vi "ASI.vi"(4 "Special Function In":string, 6 "Velocity":dbl, 7 "Abort":refnum<vi>, 8 "Axis":bool[](array[boolean]), 9 "Positions In":dbl[](array[numeric]), 10 "Action":T1=enum."MVR", 11 "VISA In":refnum<visa-resource-name>) -> (0 "Special Function Out":string, 1 "Status":bool, 2 "Position Out":dbl[](array[numeric]), 3 "VISA Out":refnum<visa-resource-name>)   [LabVIEW 2014]
uses:
  Controls/StageStates.ctl
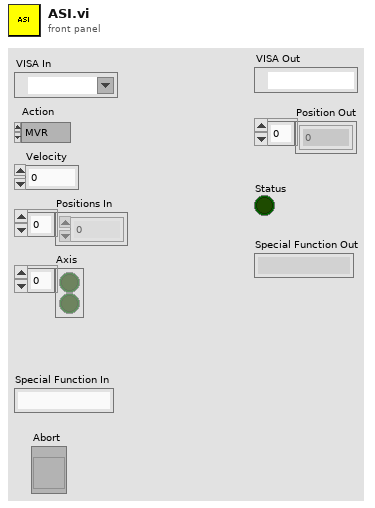
[diagram p1: front panel]
types:
  T1 = typedef "StageStates.ctl" = enum16{"POSITION", "MVR", "MOVE", "HALT", "ONTARGET", "ERROR", "EXIT", "HOME", "ZEROPOS", "NANOPOS", "QUIT", "ANALOG"}
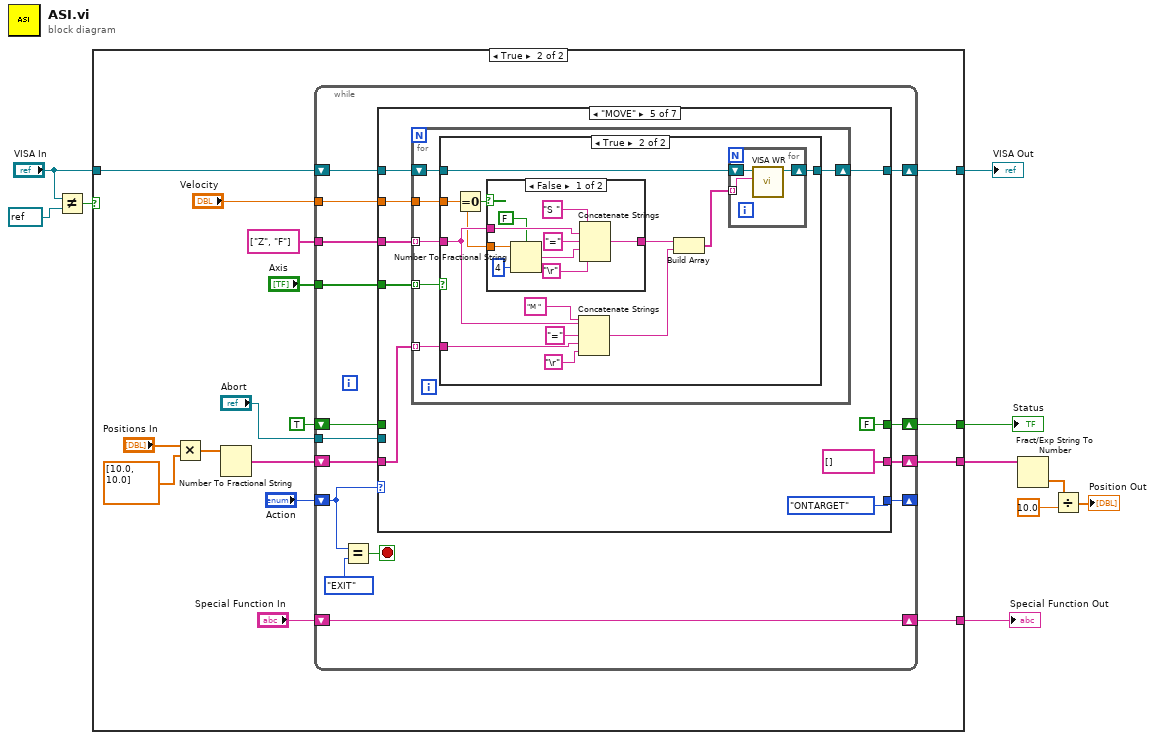
[diagram p0: block diagram]
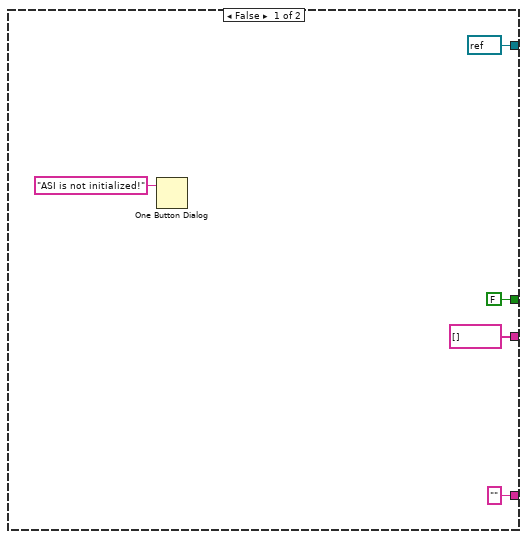
[diagram p2: hidden frame]
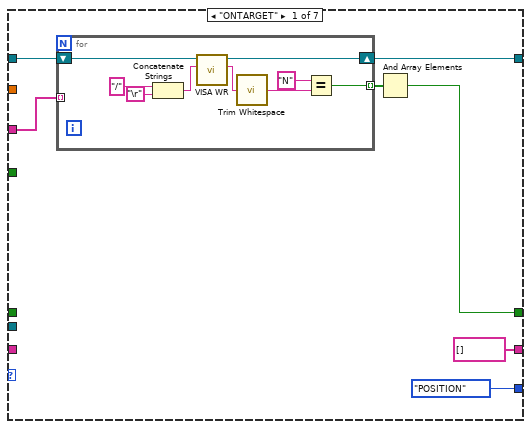
[diagram p3: hidden frame]
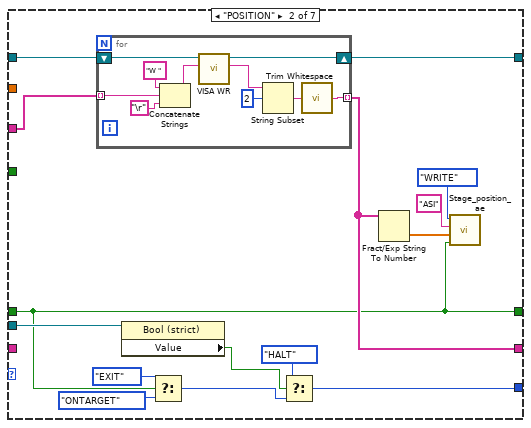
[diagram p4: hidden frame]
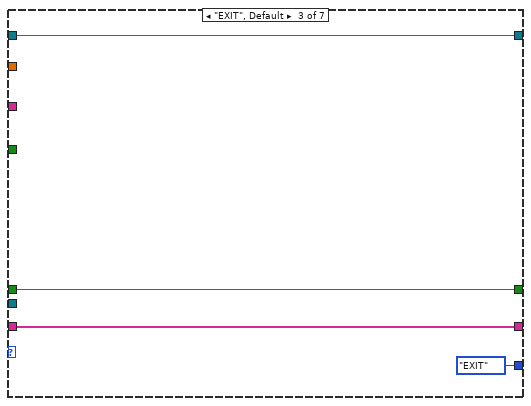
[diagram p5: hidden frame]
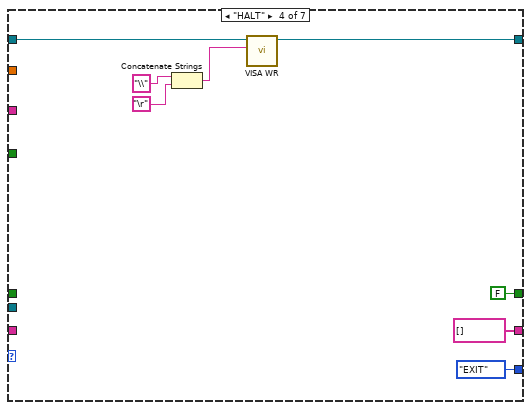
[diagram p6: hidden frame]
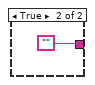
[diagram p8: hidden frame]
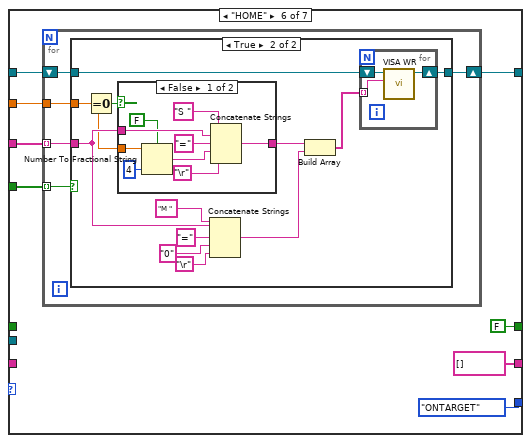
[diagram p9: hidden frame]
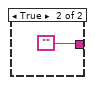
[diagram p11: hidden frame]
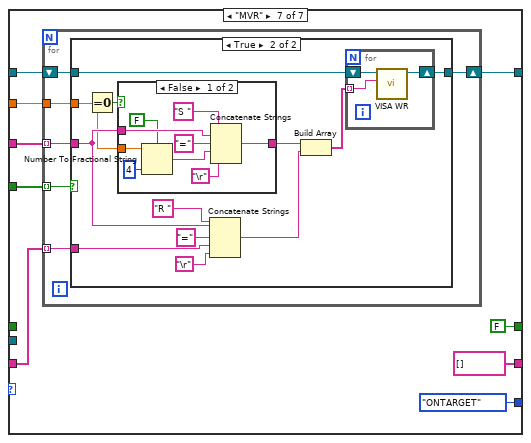
[diagram p12: hidden frame]
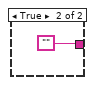
[diagram p14: hidden frame]
diagram:
  n1 = Not Equal?(x="VISA In", y=refnum<visa-resource-name> refnum ("VISA resource name")) -> (x != y?=w8:bool)
  n2 = case shown="True" w8 {
    tunnel: "VISA In" -> [_ w30]
    tunnel: [refnum<visa-resource-name> refnum ("VISA In") w23] -> w4
    tunnel: [FALSE w22] -> w3
    tunnel: [string[] [] w21] -> w2
    tunnel: ["" ("Special Function In") w20] -> w1
    frame False {
      n3 = One Button Dialog(message="ASI is not initialized!") -> ()  [unwired: 1 in, 1 out]
    }
    frame True {
      n4 = Multiply(x="Positions In", y=dbl[] [10.0, 10.0]) -> (x*y=w16:dbl[])
      n5 = Number To Fractional String(number=w16) -> (F-format string=w25:string[])  [unwired: 3 in]
      n6 = while {
        tunnel: string[] ["Z", "F"] -> [w46]
        shift-right: [w35] -> _
        shift-left: "Action" -> [w40]
        shift-right: [w43] -> w21
        shift-left: w25 -> [w44]
        shift-right: [w41] -> w22
        shift-left: TRUE -> [w42]
        tunnel: "Axis" -> [w39]
        tunnel: "Velocity" -> [w38]
        shift-right: [w37] -> w20
        shift-left: "Special Function In" -> [w37]
        shift-right: [w33] -> w23
        shift-left: w30 -> [w45]
        tunnel: "Abort" -> [w32]
        stop <- w34 stop-if-true
        n7 = Equal?(x=w40, y=StageStates."EXIT") -> (x = y?=w34:bool)
        n8 = case shown="\"MOVE\"" w40 {
          tunnel: w46 -> [w50 w76 _ _ w108 w148 w188]
          tunnel: w45 -> [w53 w77 w88 w99 w107 w147 w187]
          tunnel: w44 -> [_ _ w90 _ w106 _ w186]
          tunnel: [string[] [] w75 w90 string[] [] string[] [] string[] [] string[] []] -> w43
          tunnel: w42 -> [_ w64 w91 _ _ _ _]
          tunnel: [w51 w64 w91 FALSE FALSE FALSE FALSE] -> w41
          tunnel: w39 -> [_ _ _ _ w105 w146 w185]
          tunnel: w38 -> [_ _ _ _ w104 w145 w184]
          tunnel: [StageStates."POSITION" ("Action") w69 StageStates."EXIT" ("Action") StageStates."EXIT" ("Action") StageStates."ONTARGET" ("Action") StageStates."ONTARGET" ("Action") StageStates."ONTARGET" ("Action")] -> w35
          tunnel: [w47 w67 w88 w92 w100 w141 w180] -> w33
          tunnel: w32 -> [_ w65 _ _ _ _ _]
          frame "ONTARGET" {
            n9 = for {
              tunnel: [w58] -> w52 mode=indexing
              tunnel: w50 -> [_] mode=indexing
              shift-right: [w54] -> w47
              shift-left: w53 -> [w62]
              n10 = Concatenate Strings("/" ("string"), "\r") -> (w61:string)
              n11 = call "VISA WR.vi"("write buffer"=w61, "VISA Refnum in"=w62) -> ("read buffer"=w60:string, "VISA Refnum out"=w54:refnum<visa-resource-name>)  [unwired: 7 in, 1 out]
              n12 = call <vilib>:"Trim Whitespace.vi"("string"=w60) -> ("trimmed string"=w55:string)  [unwired: 1 in]
              n13 = Equal?(x="N", y=w55) -> (x = y?=w58:bool)
            }
            n14 = And Array Elements(Boolean array=w52) -> (logical AND=w51:bool)
          }
          frame "POSITION" {
            n15 = for {
              tunnel: [w84] -> w75 mode=indexing
              tunnel: w76 -> [w79] mode=indexing
              shift-right: [w78] -> w67
              shift-left: w77 -> [w87]
              n16 = Concatenate Strings("W " ("string"), w79, "\r") -> (w86:string)
              n17 = call "VISA WR.vi"("write buffer"=w86, "VISA Refnum in"=w87) -> ("read buffer"=w85:string, "VISA Refnum out"=w78:refnum<visa-resource-name>)  [unwired: 7 in, 1 out]
              n18 = String Subset(string=w85, offset (0)=2) -> (substring=w80:string)  [unwired: 1 in]
              n19 = call <vilib>:"Trim Whitespace.vi"("string"=w80) -> ("trimmed string"=w84:string)  [unwired: 1 in]
            }
            n20 = property class="Bool (strict)"(reference=w65) -> ("Value"=w66:bool)  [unwired: 1 in, 2 out]
            n21 = Select(t=StageStates."EXIT" ("Action"), s=w64, f=StageStates."ONTARGET" ("Action")) -> (s? t:f=w70:T1)
            n22 = Select(t=StageStates."HALT", s=w66, f=w70) -> (s? t:f=w69:T1)
            n23 = Fract/Exp String To Number(string=w75) -> (number=w63:dbl[])  [unwired: 3 in, 1 out]
            n24 = call "Stage_position_ae.vi"("Status In"=w64, "Position In"=w63, "StageID"="ASI", "Enum"=enum16{"WRITE", "READ"}."WRITE") -> ()  [unwired: 6 in, 2 out]
          }
          frame "EXIT", Default {
          }
          frame "HALT" {
            n25 = Concatenate Strings("\\" ("string"), "\r") -> (w95:string)
            n26 = call "VISA WR.vi"("write buffer"=w95, "VISA Refnum in"=w99) -> ("VISA Refnum out"=w92:refnum<visa-resource-name>)  [unwired: 7 in, 2 out]
          }
          frame "MOVE" {
            n27 = for {
              tunnel: w108 -> [w114] mode=indexing
              tunnel: w106 -> [w113] mode=indexing
              shift-right: [w111] -> w100
              shift-left: w107 -> [w112]
              tunnel: w105 -> [w110] mode=indexing
              tunnel: w104 -> [w109]
              n28 = case shown="True" w110 {
                tunnel: w114 -> [_ w121]
                tunnel: w113 -> [_ w124]
                tunnel: w112 -> [w115 w123]
                tunnel: [w115 w122] -> w111
                tunnel: w109 -> [_ w120]
                frame False {
                }
                frame True {
                  n29 = Equal To 0?(x=w120) -> (x = 0?=w119:bool)
                  n30 = case shown="False" w119 {
                    tunnel: w121 -> [w136 _]
                    tunnel: w120 -> [w133 _]
                    tunnel: [w135 ""] -> w118
                    frame False {
                      n31 = Number To Fractional String(use system decimal point (T)=FALSE, number=w133, precision (6)=i16 4) -> (F-format string=w134:string)  [unwired: 1 in]
                      n32 = Concatenate Strings("S ", w136, "=", w134, "\r") -> (w135:string)
                    }
                    frame True {
                    }
                  }
                  n33 = Concatenate Strings("M ", w121, "=", w124, "\r") -> (w117:string)
                  n34 = Build Array(w118, w117) -> (w116:string[])
                  n35 = for {
                    shift-right: [w129] -> w122
                    shift-left: w123 -> [w130]
                    tunnel: w116 -> [w128] mode=indexing
                    n36 = call "VISA WR.vi"("write buffer"=w128, "VISA Refnum in"=w130) -> ("VISA Refnum out"=w129:refnum<visa-resource-name>)  [unwired: 7 in, 2 out]
                  }
                }
              }
            }
          }
          frame "HOME" {
            n37 = for {
              tunnel: w148 -> [w153] mode=indexing
              shift-right: [w151] -> w141
              shift-left: w147 -> [w152]
              tunnel: w146 -> [w150] mode=indexing
              tunnel: w145 -> [w149]
              n38 = case shown="True" w150 {
                tunnel: w153 -> [_ w161]
                tunnel: w152 -> [w154 w163]
                tunnel: [w154 w162] -> w151
                tunnel: w149 -> [_ w160]
                frame False {
                }
                frame True {
                  n39 = Equal To 0?(x=w160) -> (x = 0?=w159:bool)
                  n40 = case shown="False" w159 {
                    tunnel: w161 -> [w175 _]
                    tunnel: w160 -> [w172 _]
                    tunnel: [w174 ""] -> w158
                    frame False {
                      n41 = Number To Fractional String(use system decimal point (T)=FALSE, number=w172, precision (6)=i16 4) -> (F-format string=w173:string)  [unwired: 1 in]
                      n42 = Concatenate Strings("S ", w175, "=", w173, "\r") -> (w174:string)
                    }
                    frame True {
                    }
                  }
                  n43 = Concatenate Strings("M ", w161, "=", "0" ("string"), "\r") -> (w157:string)
                  n44 = Build Array(w158, w157) -> (w156:string[])
                  n45 = for {
                    shift-right: [w168] -> w162
                    shift-left: w163 -> [w169]
                    tunnel: w156 -> [w167] mode=indexing
                    n46 = call "VISA WR.vi"("write buffer"=w167, "VISA Refnum in"=w169) -> ("VISA Refnum out"=w168:refnum<visa-resource-name>)  [unwired: 7 in, 2 out]
                  }
                }
              }
            }
          }
          frame "MVR" {
            n47 = for {
              tunnel: w188 -> [w194] mode=indexing
              tunnel: w186 -> [w193] mode=indexing
              shift-right: [w191] -> w180
              shift-left: w187 -> [w192]
              tunnel: w185 -> [w190] mode=indexing
              tunnel: w184 -> [w189]
              n48 = case shown="True" w190 {
                tunnel: w194 -> [_ w201]
                tunnel: w193 -> [_ w204]
                tunnel: w192 -> [w195 w203]
                tunnel: [w195 w202] -> w191
                tunnel: w189 -> [_ w200]
                frame False {
                }
                frame True {
                  n49 = Equal To 0?(x=w200) -> (x = 0?=w199:bool)
                  n50 = case shown="False" w199 {
                    tunnel: w201 -> [w216 _]
                    tunnel: w200 -> [w214 _]
                    tunnel: [w215 ""] -> w198
                    frame False {
                      n51 = Number To Fractional String(use system decimal point (T)=FALSE, number=w214, precision (6)=i16 4) -> (F-format string=w213:string)  [unwired: 1 in]
                      n52 = Concatenate Strings("S ", w216, "=", w213, "\r") -> (w215:string)
                    }
                    frame True {
                    }
                  }
                  n53 = Concatenate Strings("R ", w201, "=", w204, "\r") -> (w197:string)
                  n54 = Build Array(w198, w197) -> (w196:string[])
                  n55 = for {
                    shift-right: [w209] -> w202
                    shift-left: w203 -> [w210]
                    tunnel: w196 -> [w208] mode=indexing
                    n56 = call "VISA WR.vi"("write buffer"=w208, "VISA Refnum in"=w210) -> ("VISA Refnum out"=w209:refnum<visa-resource-name>)  [unwired: 7 in, 2 out]
                  }
                }
              }
            }
          }
        }
      }
    }
  }
  "Status" <- w3
  "Special Function Out" <- w1
  "VISA Out" <- w4
  n57 = Fract/Exp String To Number(string=w2) -> (number=w6:dbl[])  [unwired: 3 in, 1 out]
  n58 = Divide(x=w6, y=10.0) -> (x/y=→"Position Out":dbl[])
